vi "Densidade de Probabilidade e Confiailidade.vi"() -> ()   [LabVIEW 2020]
uses:
  <vilib>/Analysis/NI_AALPro.lvlib
panel:
  in  "Tabelas":i32[](listbox)
  out "Confiability":cluster{"Ramp Pattern":dbl[], dbl[]}(graph)
  out "Waveform Graph":dbl[](graph)
  out "Histogram Graph":cluster{"Axis":dbl[], "Histogram":i32[]}(graph)
  out "Cumulative Density Function (CDF)":cluster{"Ramp Pattern":dbl[], dbl[]}(graph)
  out "Probability Density Function (PDF)":cluster{"Ramp Pattern":dbl[], dbl[]}(graph)
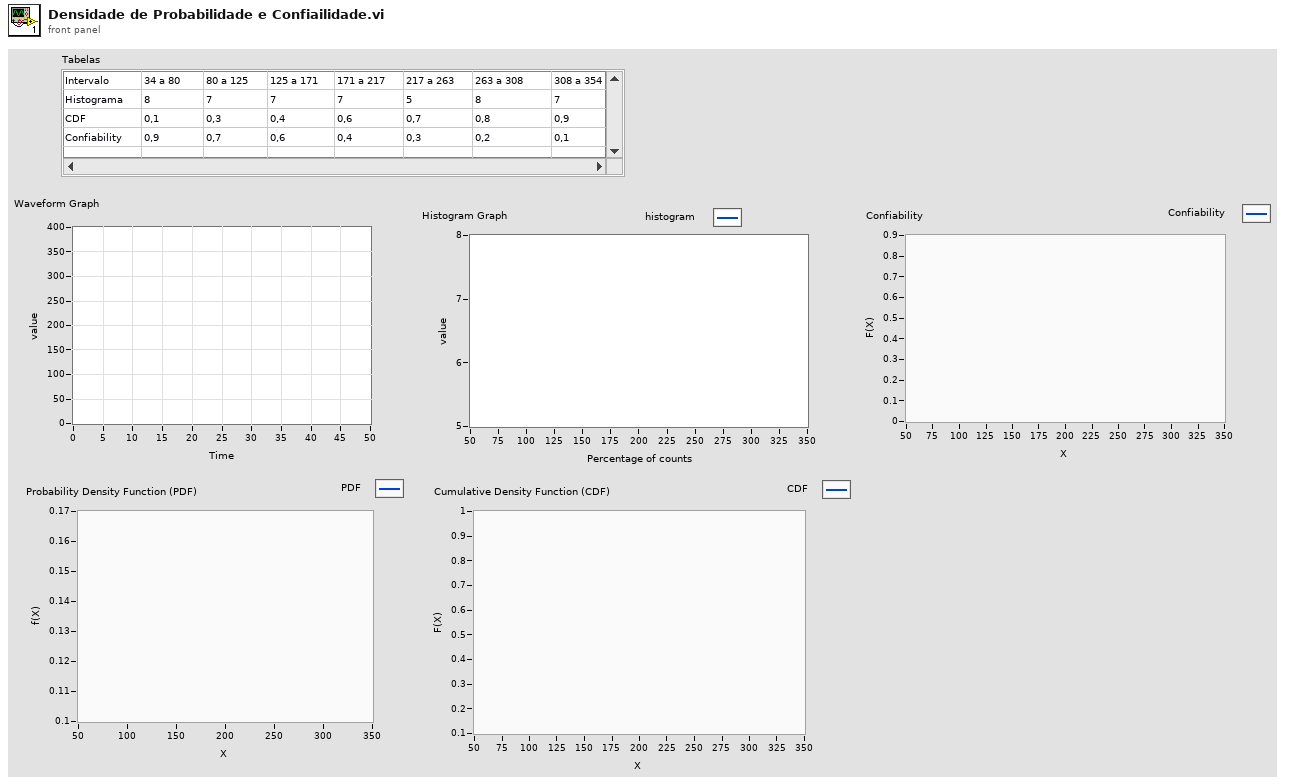
[diagram p1: front panel]
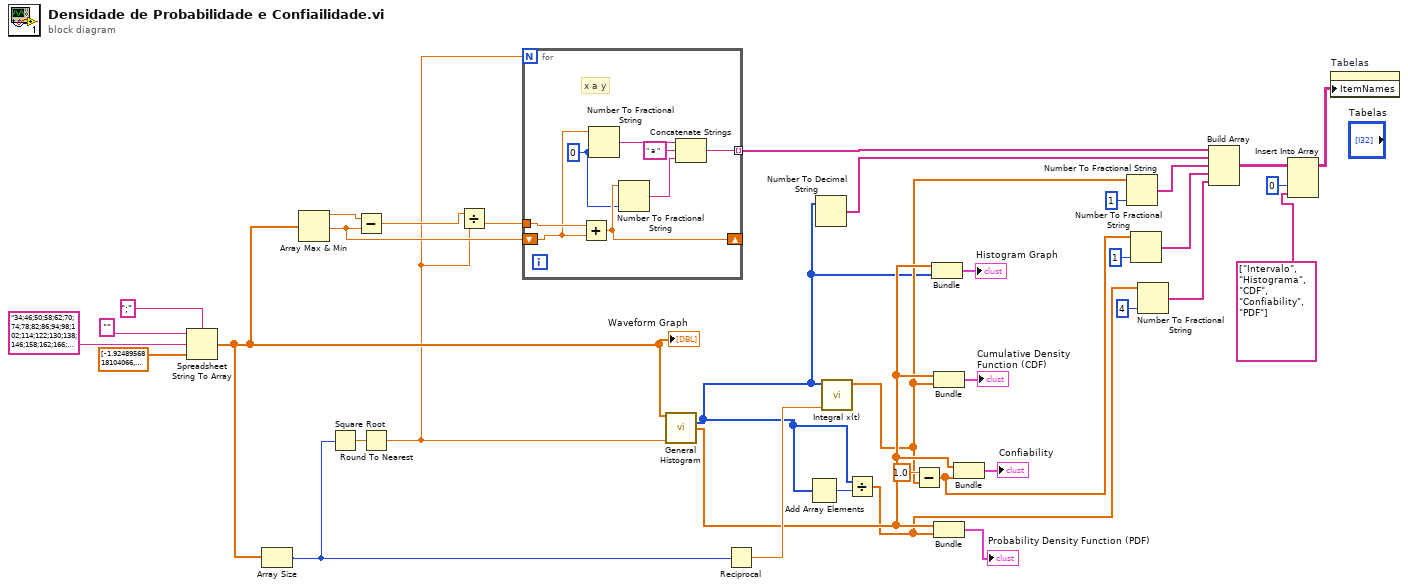
[diagram p0: block diagram]
diagram:
  n1 = Spreadsheet String To Array(delimiter (Tab)=";", format string="", spreadsheet string="34;46;50;58;62;70;74;78;82;86;94;98;102;114;122;130;138;146;158;162;166;170;174;186;190;194;198;210;214;226;230;234;246;254;270;282;286;290;294;298;302;306;310;326;330;334;338;342;354", array type (2D Dbl)=dbl[] [-1.9248956818104066, 0.3112342515348463, 1.8692362658018304, -0.5776880888424503, 0.20934604621485975, 1.4475109318963486, 0.7675061953982794, -0.218373425372552, 1.355879072392087, -0.6031761167957952, 0.2848639300682354, -0.4523629840942558, 0.39309206576819067, -1.1131811654833368, 1.1008781459025572, -0.7187890386395429, -0.3261549911479751, 1.0591757017035908, 0.3805091962850973, 0.18837332728848377, 0.48334639809867275, 0.6734791628214536, -2.446547973674908, -0.6938822322242062, -1.126964642802215, 0.8740199282566117, 1.0482087685313595, 0.6623549447079551, -0.5794262846897151, 1.424863822052554, -1.3945761742114473, 0.07772457073479355, 0.9886746146176917, 0.38117909489292523, -1.007011015166027, -1.769139934462521, 0.17311443430858997, -0.055235020387792044, 1.2821181406845978, 0.14918495038348412, -0.7469973627119986, -0.02371599756363585, 0.6556605065090322, 0.07512361421046454, 1.7510040225711374, -0.9696567696479239, 0.06720607690029623, -1.1391189041401273, -0.45398607765088883, -0.033604298177246195] ("Waveform Graph")) -> (array=w24:dbl[])
  "Waveform Graph" <- w24
  n2 = Array Size(array=w24) -> (size(s)=w30:i32)
  n3 = Array Max & Min(array=w24) -> (max value=w23:dbl, min value=w22:dbl)  [unwired: 2 out]
  n4 = Square Root(x=w30) -> (sqrt(x)=w29:dbl)
  n5 = Subtract(x=w23, y=w22) -> (x-y=w18:dbl)
  n6 = Round To Nearest(number=w29) -> (nearest integer value=w17:dbl)
  n7 = Divide(x=w18, y=w17) -> (x/y=w19:dbl)
  n8 = for {
    N: w17 -> [_]
    tunnel: w19 -> [w44]
    shift-right: [w42] -> _
    shift-left: w22 -> [w43]
    tunnel: [w38] -> w21 mode=indexing
    w37 = i16 0 ("precision (6)")
    # "x a y"
    n9 = Add(x=w44, y=w43) -> (x+y=w42:dbl)
    n10 = Number To Fractional String(number=w43, precision (6)=w37) -> (F-format string=w41:string)  [unwired: 2 in]
    n11 = Number To Fractional String(number=w42, precision (6)=w37) -> (F-format string=w39:string)  [unwired: 2 in]
    n12 = Concatenate Strings(w41, " a " ("string"), w39) -> (w38:string)
  }
  n13 = call <vilib>:"General Histogram.vi"("X"=w24, "# bins"=w17) -> ("Histogram"=w7:i32[], "Axis"=w25:dbl[])  [unwired: 9 in, 3 out]
  n14 = Reciprocal(x=w30) -> (1/x=w28:dbl)
  n15 = Add Array Elements(numeric array=w7) -> (sum=w8:i32)
  n16 = Number To Decimal String(number=w7) -> (decimal integer string=w20:string[])  [unwired: 1 in]
  n17 = call <vilib>:"Integral x(t).vi"("dt"=w28, "X"=w7) -> ("Integral X"=w15:dbl[])  [unwired: 8 in, 1 out]
  n18 = Divide(x=w7, y=w8) -> (x/y=w5:dbl[])
  n19 = Subtract(x=1.0, y=w15) -> (x-y=w12:dbl[])
  n20 = Bundle("Axis"=w25, "Histogram"=w7) -> (→"Histogram Graph":cluster{"Axis":dbl[], "Histogram":i32[]})  [unwired: 1 in]
  n21 = Bundle("Axis"=w25, "Integral X"=w15) -> (→"Cumulative Density Function (CDF)":cluster{"Axis":dbl[], "Integral X":dbl[]})  [unwired: 1 in]
  n22 = Bundle("Axis"=w25, w5) -> (→"Probability Density Function (PDF)":cluster{"Axis":dbl[], dbl[]})  [unwired: 1 in]
  n23 = Bundle("Axis"=w25, w12) -> (→"Confiability":cluster{"Axis":dbl[], dbl[]})  [unwired: 1 in]
  n24 = Number To Fractional String(number=w15, precision (6)=i16 1) -> (F-format string=w14:string[])  [unwired: 2 in]
  n25 = Number To Fractional String(number=w12, precision (6)=i16 1) -> (F-format string=w11:string[])  [unwired: 2 in]
  n26 = Number To Fractional String(number=w5, precision (6)=i16 4) -> (F-format string=w9:string[])  [unwired: 2 in]
  n27 = Build Array(w21, w20, w14, w11, w9) -> (w4:string[][])
  n28 = Insert Into Array(array=w4, index (col)=0 ("disabled index (col)"), new element=string[] ["Intervalo", "Histograma", "CDF", "Confiability", "PDF"]) -> (w1:string[][])  [unwired: 1 in]
  n29 = property on="Tabelas" class="MCListbox (strict)"("ItemNames"=w1) -> ()  [unwired: 2 in, 2 out]
